vi "关闭采集卡.vi"(11 "error in":errorcluster caption="错误输入") -> (3 "error out":errorcluster caption="错误输出")   [LabVIEW 2016]
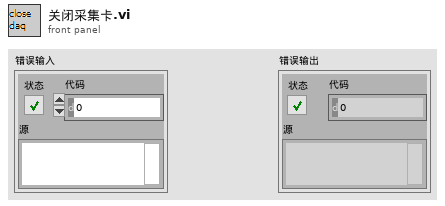
[diagram p1: front panel]
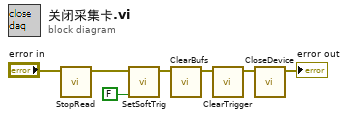
[diagram p0: block diagram]
diagram:
  n1 = call "StopRead.vi"("error in"="error in") -> ("error out"=w5:errorcluster)  [unwired: 10 in]
  n2 = call "SetSoftTrig.vi"("SoftTrig"=FALSE, "error in"=w5) -> ("error out"=w4:errorcluster)  [unwired: 9 in]
  n3 = call "ClearBufs.vi"("error in"=w4) -> ("error out"=w2:errorcluster)  [unwired: 10 in]
  n4 = call "ClearTrigger.vi"("错误输入（无错误）"=w2) -> ("错误输出"=w1:errorcluster)  [unwired: 10 in]
  n5 = call "CloseDevice.vi"("error in"=w1) -> ("error out"=→"error out":errorcluster)  [unwired: 10 in]
